vi "FTW-Actor-UnknownJob.vi"(0 "FTW Actor Instance":refnum<class "FTW-ActorInstance.lvclass">, 5 "Unknown Job":string, 11 "error in":errorcluster) -> (4 "FTW Actor Instance out":refnum<class "FTW-ActorInstance.lvclass">, 15 "error out":errorcluster)   [LabVIEW 2013, in "FTW-Actor.lvlib" / "FTW-ActorInstance.lvclass"]
uses:
  FTW-ActorInstance.lvclass
panel:
  # "Inputs"
  # "Outputs"
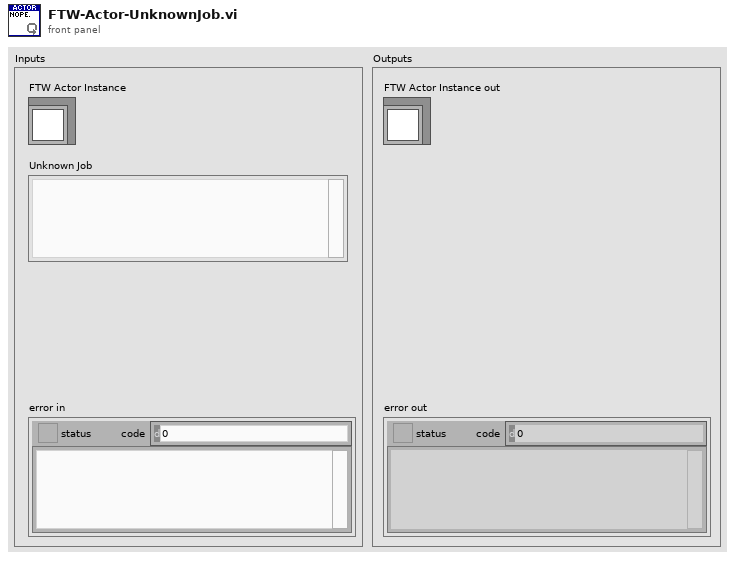
[diagram p1: front panel]
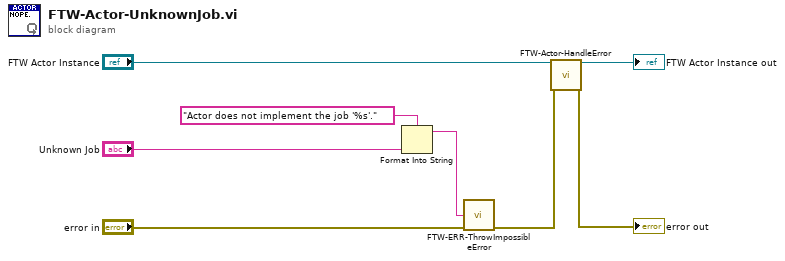
[diagram p0: block diagram]
diagram:
  n1 = Format Into String(format string="Actor does not implement the job '%s'.", "Unknown Job") -> (resulting string=w7:string)  [unwired: 2 in, 1 out]
  n2 = call "FTW-ERR-ThrowImpossibleError.vi"("Reason this error should never happen"=w7, "error in"="error in") -> ("error out"=w2:errorcluster)  [unwired: 13 in]
  n3 = call-dynamic "FTW-Actor-HandleError.vi"("FTW Actor Instance"="FTW Actor Instance", "error in"=w2) -> ("FTW Actor Instance out"=→"FTW Actor Instance out":refnum<class "FTW-ActorInstance.lvclass">, "error out"=→"error out":errorcluster)  [unwired: 11 in, 1 out]
